vi "getHorizontalSettingsFromHW.vi"(8 "error in (no error)":errorcluster, 11 "TektronixDPO in":refnum<class "TektronixDPO.lvclass">) -> (0 "error out":errorcluster, 3 "TektronixDPO out":refnum<class "TektronixDPO.lvclass">)   [LabVIEW 2013, in "TektronixDPO.lvclass"]
uses:
  TektronixDPO.lvclass
  TektronixDPO.lvclass/TektronixDPO.ctl
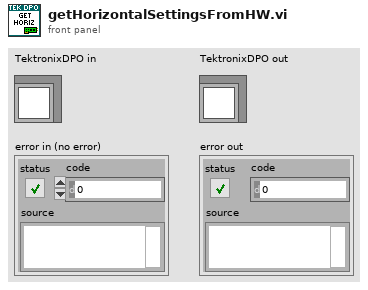
[diagram p1: front panel]
types:
  T1 = typedef "Choice77.ctl" = enum16{"1E+3", "10E+3", "100E+3", "1E+6", "5E+6", "10E+6"}
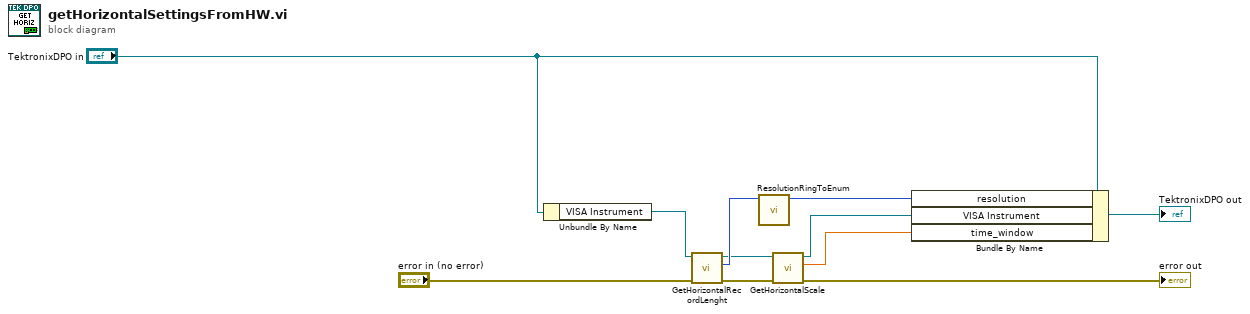
[diagram p0: block diagram]
diagram:
  n1 = Unbundle By Name("TektronixDPO in") -> ("VISA Instrument"=w11:refnum<visa-resource-name>)
  n2 = call "GetHorizontalRecordLenght.vi"("error in (no error)"="error in (no error)", "VISA Refnum in"=w11) -> ("error out"=w3:errorcluster, "Resolution"=w8:u32, "VISA Refnum out"=w4:refnum<visa-resource-name>)  [unwired: 7 in]
  n3 = call "ResolutionRingToEnum.vi"("Resolution(Enum)"=w8) -> ("Resolution(Ring)"=w9:T1)  [unwired: 10 in]
  n4 = call "GetHorizontalScale.vi"("error in (no error)"=w3, "VISA Refnum in"=w4) -> ("error out"=→"error out":errorcluster, "HorizontalScale(sec)"=w5:dbl, "VISA Refnum out"=w7:refnum<visa-resource-name>)  [unwired: 7 in]
  n5 = Bundle By Name(cluster="TektronixDPO in", "resolution"=w9, "VISA Instrument"=w7, "time_window"=w5) -> (→"TektronixDPO out":refnum<class "TektronixDPO.lvclass">)
